vi "Init.vi"(8 "error in":errorcluster, 11 "Session":T1="cam0") -> (0 "error out  - closing camera":errorcluster, 1 "error out":errorcluster, 2 "Success?":bool, 3 "IMAQdx Session OUT":T1, 4 "Gain - READ":dbl, 5 "Message":string, 6 "Exposure Time - READ":dbl, 7 "Device Serial Number":string)   [LabVIEW 2014]
uses:
  <vilib>/userdefined/High Color/IMAQdx.ctl
  <vilib>/vision/driver/IMAQdx.llb/IMAQdx Camera Control Mode.ctl
  <vilib>/vision/driver/IMAQdx.llb/IMAQdx Acquisition Mode.ctl
  <vilib>/vision/driver/NI_Vision_Acquisition_Software.lvlib
  <resource>/objmgr/imaqdx.rc
panel:
  out "ModelName":string
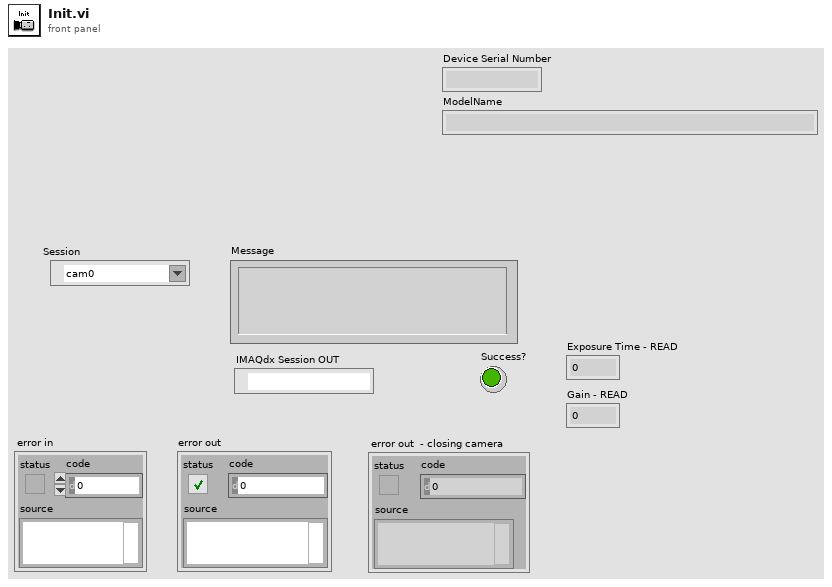
[diagram p1: front panel]
types:
  T1 = typedef "IMAQdx.ctl" = refnum<k21>
  T2 = typedef "NI_Vision_Acquisition_Software.lvlib/IMAQdx Camera Control Mode.ctl" = enum32{"Controller", "Listener"}
  T3 = typedef "NI_Vision_Acquisition_Software.lvlib/IMAQdx Acquisition Mode.ctl" = enum32{"One Shot", "Continuous"}
  T4 = cluster{"Type":u32, "Version":u32, "Flags":u32, "SerialNumberHigh":u32, "SerialNumberLow":u32, "BusType":u32, "InterfaceName":string, "VendorName":string, "ModelName":string, "CameraFileName":string, "CameraAttributeURL":string}[]
  T5 = typedef "NI_Vision_Acquisition_Software.lvlib/IMAQdx Attribute Type.ctl" = enum32{"U32", "I64", "DBL", "String", "Enum", "Bool", "Command"}
  T6 = cluster{"Attribute Type":T5, "Readable":bool, "Writable":bool, "Attribute Name":string}[]
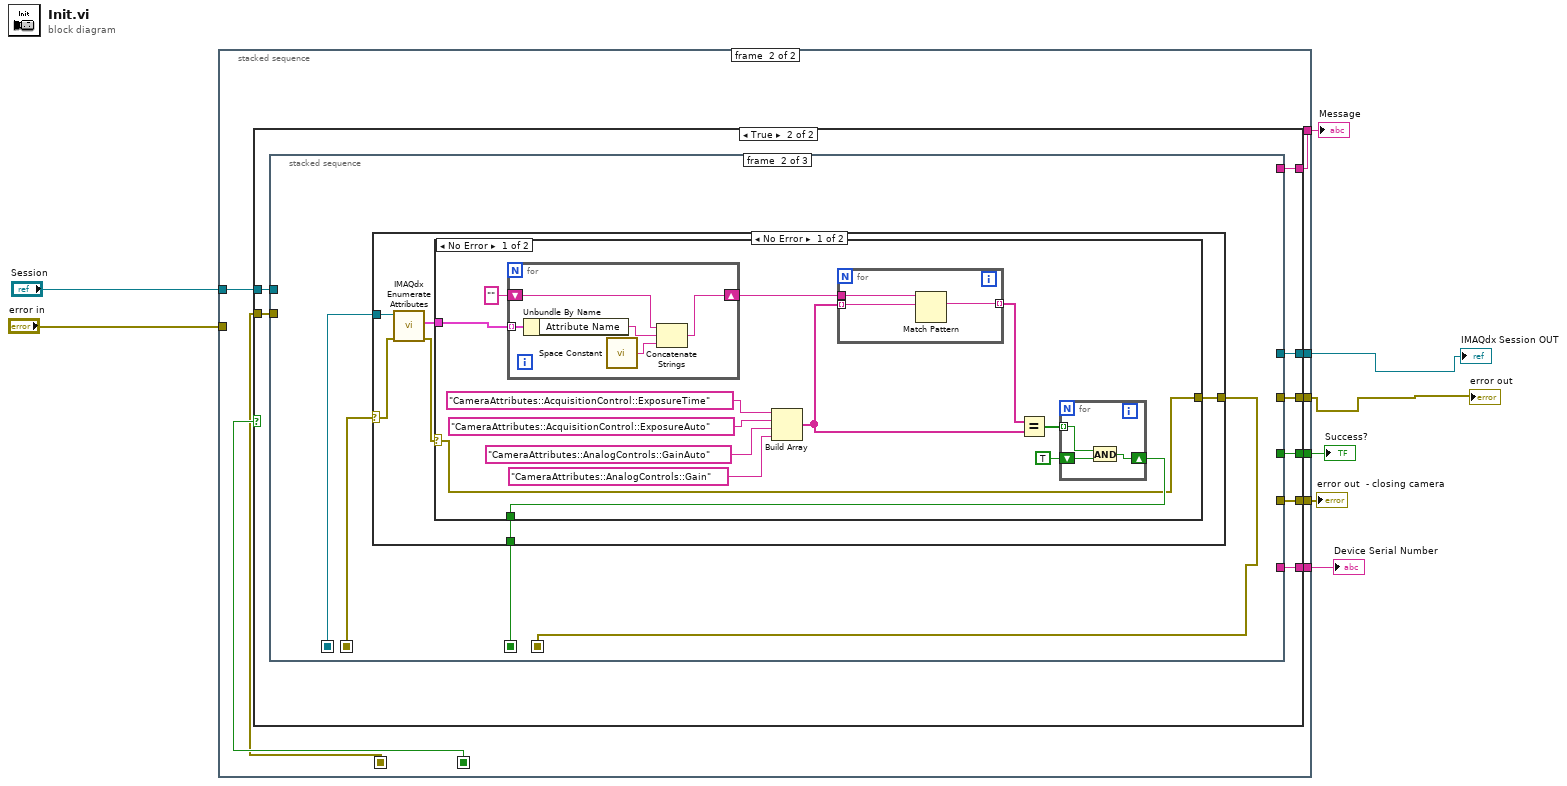
[diagram p0: block diagram]
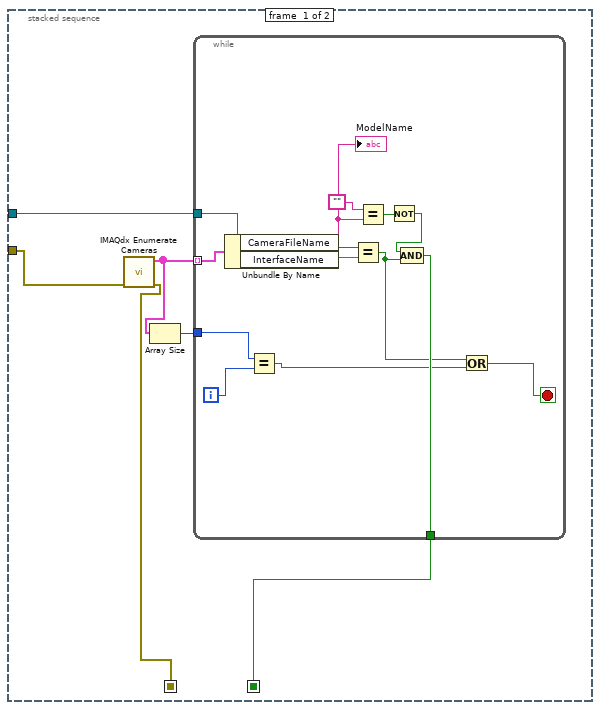
[diagram p2: hidden frame]
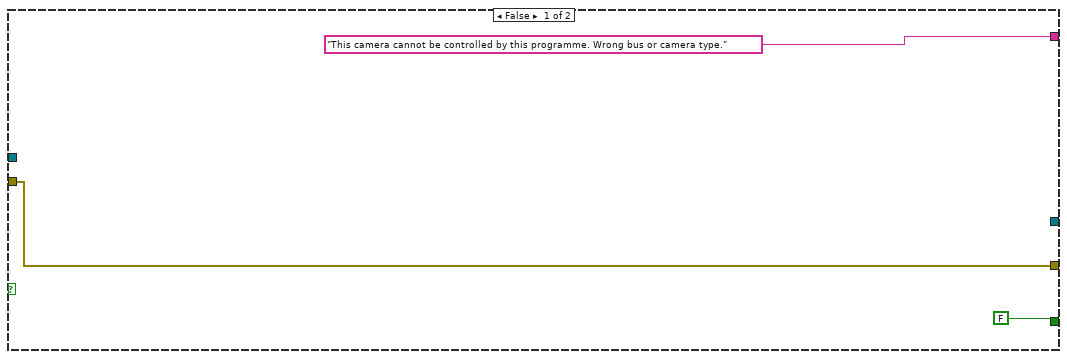
[diagram p3: hidden frame]
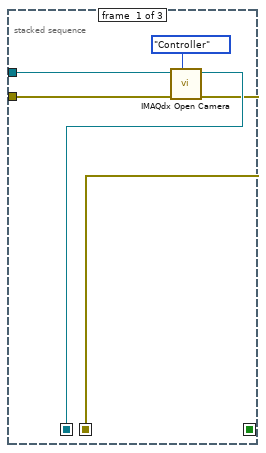
[diagram p4: hidden frame]
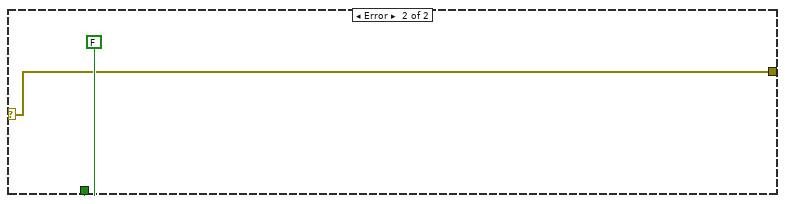
[diagram p5: hidden frame]
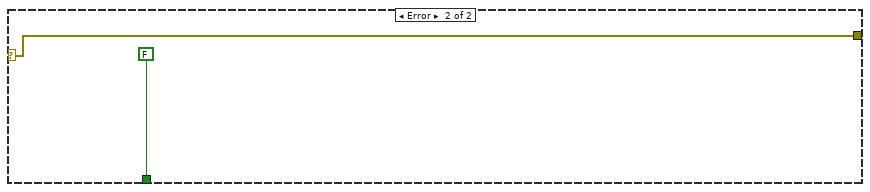
[diagram p6: hidden frame]
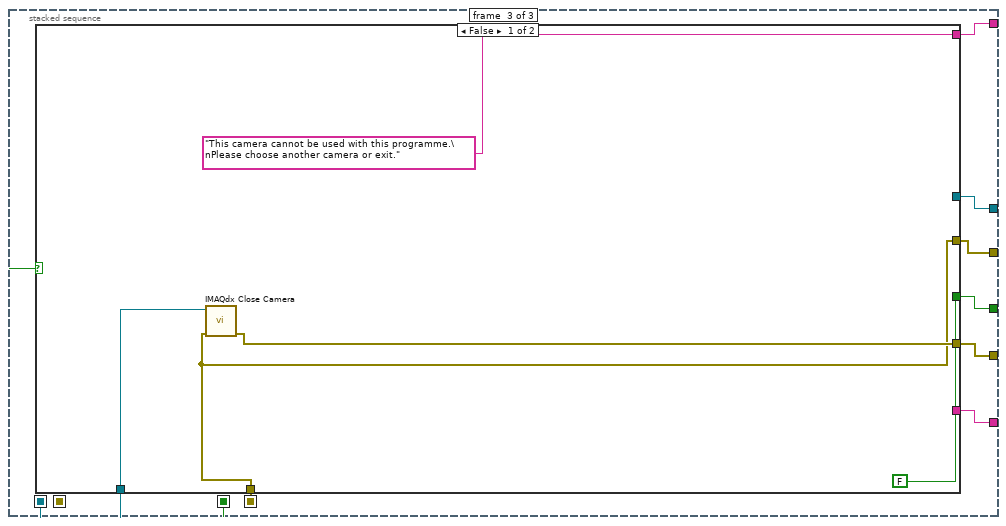
[diagram p7: hidden frame]
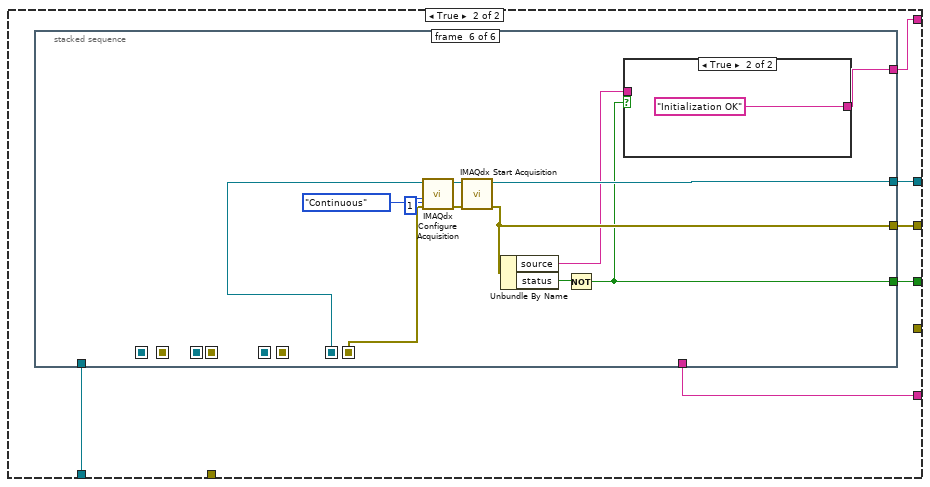
[diagram p8: hidden frame]
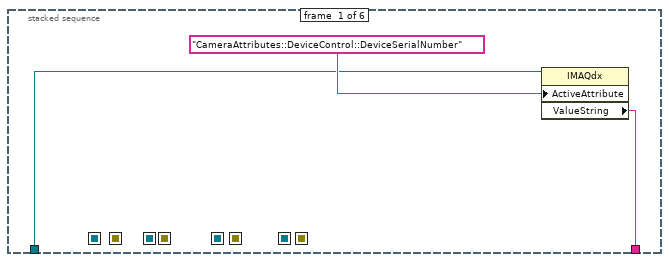
[diagram p9: hidden frame]
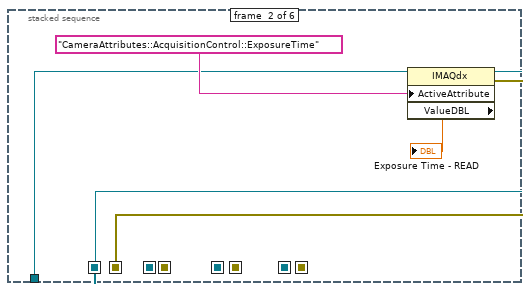
[diagram p10: hidden frame]
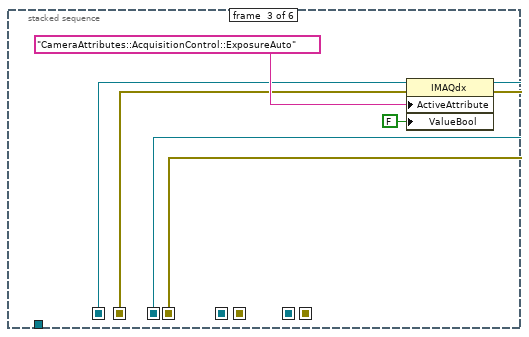
[diagram p11: hidden frame]
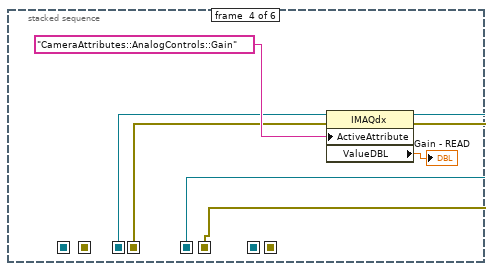
[diagram p12: hidden frame]
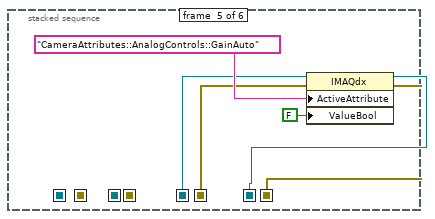
[diagram p13: hidden frame]
diagram:
  n1 = stacked-sequence {
    seq-local: [w13 _] -> [_ w31]
    seq-local: [w9 _] -> [_ w28]
    tunnel: [_ w36] -> w8
    tunnel: [_ w35] -> w2
    tunnel: [_ w30] -> w1
    tunnel: [_ w34] -> w7
    tunnel: "Session" -> [w14 w33]
    tunnel: [_ w32] -> w5
    tunnel: "error in" -> [w10 _]
    tunnel: [_ w29] -> w3
    frame #0 {
      n2 = call <vilib>:"IMAQdx Enumerate Cameras.vi"("error in"=w10) -> ("error out"=w9:errorcluster, "Camera Information Array"=w12:T4)  [unwired: 9 in]
      n3 = Array Size(array=w12) -> (size(s)=w11:i32)
      n4 = while {
        tunnel: w12 -> [w27] mode=indexing
        tunnel: w14 -> [w26]
        tunnel: [w22] -> w13
        tunnel: w11 -> [w23]
        i -> [w24]
        stop <- w20 stop-if-true
        n5 = Unbundle By Name(w27) -> ("CameraFileName"=w19:string, "InterfaceName"=w25:string)
        "ModelName" <- w19
        n6 = Equal?(x=w23, y=w24) -> (x = y?=w21:bool)
        n7 = Equal?(x=w26, y=w25) -> (x = y?=w15:bool)
        n8 = Equal?(x="", y=w19) -> (x = y?=w17:bool)
        n9 = Not(x=w17) -> (.not. x?=w16:bool)
        n10 = Compound Arithmetic op=AND(w16, w15) -> (w22:bool)
        n11 = Or(x=w15, y=w21) -> (x .or. y?=w20:bool)
      }
    }
    frame #1 {
      n12 = case shown="True" w31 {
        tunnel: ["This camera cannot be controlled by this programme. Wrong bus or camera type." ("source") w47] -> w36
        tunnel: [_ w46] -> w35
        tunnel: [FALSE w45] -> w34
        tunnel: w33 -> [_ w44]
        tunnel: [_ w43] -> w32
        tunnel: w28 -> [w38 w42]
        tunnel: [w38 w40] -> w30
        tunnel: [_ w41] -> w29
        frame False {
        }
        frame True {
          n13 = stacked-sequence {
            seq-local: [w50 _ _] -> [_ w54 _]
            seq-local: [w51 _ _] -> [_ w56 w99]
            seq-local: [_ w55 _] -> [_ _ w98]
            seq-local: [_ w53 _] -> [_ _ w92]
            tunnel: [_ _ w97] -> w47
            tunnel: [_ _ w96] -> w46
            tunnel: [_ _ w95] -> w45
            tunnel: w44 -> [w49 _ _]
            tunnel: [_ _ w94] -> w43
            tunnel: w42 -> [w48 _ _]
            tunnel: [_ _ w93] -> w41
            tunnel: [_ _ w91] -> w40
            frame #0 {
              n14 = call <vilib>:"IMAQdx Open Camera.vi"("Camera Control Mode"=IMAQdx_Camera_Control_Mode."Controller", "error in"=w48, "Session In"=w49) -> ("error out"=w50:errorcluster, "Session Out"=w51:T1)  [unwired: 7 in]
            }
            frame #1 {
              n15 = case shown="No Error" w54 {
                selector: w54 -> [w58 w89]
                tunnel: w56 -> [w62 _]
                tunnel: [w60 FALSE] -> w55
                tunnel: [w57 w89] -> w53
                frame No Error {
                  n16 = call <vilib>:"IMAQdx Enumerate Attributes.vi"("error in"=w58, "Session In"=w62) -> ("error out"=w59:errorcluster, "Attribute Information Array"=w61:T6)  [unwired: 7 in, 1 out]
                  n17 = case shown="No Error" w59 {
                    selector: w59 -> [w63 w87]
                    tunnel: w61 -> [w75 _]
                    tunnel: [w65 FALSE] -> w60
                    tunnel: [w63 w87] -> w57
                    frame No Error {
                      n18 = for {
                        tunnel: w75 -> [w86] mode=indexing
                        shift-right: [w83] -> w69
                        shift-left: "" -> [w82]
                        n19 = Unbundle By Name(w86) -> ("Attribute Name"=w85:string)
                        n20 = call <vilib>:"Space Constant.vi"() -> ("String"=w84:string)
                        n21 = Concatenate Strings(w82, w85, w84) -> (w83:string)
                      }
                      n22 = Build Array("CameraAttributes::AcquisitionControl::ExposureTime" ("Attribute Name"), "CameraAttributes::AcquisitionControl::ExposureAuto" ("Attribute Name"), "CameraAttributes::AnalogControls::GainAuto" ("Attribute Name"), "CameraAttributes::AnalogControls::Gain" ("Attribute Name")) -> (w64:string[])
                      n23 = for {
                        tunnel: w69 -> [w81]
                        tunnel: w64 -> [w80] mode=indexing
                        tunnel: [w79] -> w68 mode=indexing
                        n24 = Match Pattern(string=w81, regular expression=w80) -> (match substring=w79:string)  [unwired: 1 in, 3 out]
                      }
                      n25 = Equal?(x=w68, y=w64) -> (x = y?=w67:bool[])
                      n26 = for {
                        tunnel: w67 -> [w78] mode=indexing
                        shift-right: [w76] -> w65
                        shift-left: TRUE -> [w77]
                        n27 = And(x=w78, y=w77) -> (x .and. y?=w76:bool)
                      }
                    }
                    frame Error {
                    }
                  }
                }
                frame Error {
                }
              }
            }
            frame #2 {
              n28 = case shown="False" w98 {
                tunnel: w99 -> [w104 w110]
                tunnel: ["This camera cannot be used with this programme.\nPlease choose another camera or exit." w106] -> w97
                tunnel: [_ w109] -> w96
                tunnel: [w100 w108] -> w91
                tunnel: [FALSE w107] -> w95
                tunnel: [w101 _] -> w94
                tunnel: [_ w105] -> w93
                tunnel: w92 -> [w100 _]
                frame False {
                  n29 = call <vilib>:"IMAQdx Close Camera.vi"("error in"=w100, "Session In"=w104) -> ("error out"=w101:errorcluster)  [unwired: 9 in]
                }
                frame True {
                  n30 = stacked-sequence {
                    seq-local: [_ w115 _ _ _ _] -> [_ _ w121 _ _ _]
                    seq-local: [_ w114 _ _ _ _] -> [_ _ w122 _ _ _]
                    seq-local: [_ _ w120 _ _ _] -> [_ _ _ w128 _ _]
                    seq-local: [_ _ w119 _ _ _] -> [_ _ _ w127 _ _]
                    seq-local: [_ _ _ w126 _ _] -> [_ _ _ _ w134 _]
                    seq-local: [_ _ _ w125 _ _] -> [_ _ _ _ w133 _]
                    seq-local: [_ _ _ _ w132 _] -> [_ _ _ _ _ w141]
                    seq-local: [_ _ _ _ w131 _] -> [_ _ _ _ _ w140]
                    tunnel: w110 -> [w112 w117 _ _ _ _]
                    tunnel: [_ _ _ _ _ w144] -> w109
                    tunnel: [_ _ _ _ _ w143] -> w108
                    tunnel: [_ _ _ _ _ w139] -> w107
                    tunnel: [_ _ _ _ _ w138] -> w106
                    tunnel: [w111 _ _ _ _ _] -> w105
                    frame #0 {
                      n31 = property class="IMAQdx"(reference=w112, "ActiveAttribute"="CameraAttributes::DeviceControl::DeviceSerialNumber" ("Attribute Name")) -> ("ValueString"=w111:string)  [unwired: 1 in, 2 out]
                    }
                    frame #1 {
                      n32 = property class="IMAQdx"(reference=w117, "ActiveAttribute"="CameraAttributes::AcquisitionControl::ExposureTime" ("Attribute Name")) -> (reference out=w114:T1, error out=w115:errorcluster, "ValueDBL"=→"Exposure Time - READ":dbl)  [unwired: 1 in]
                    }
                    frame #2 {
                      n33 = property class="IMAQdx"(reference=w122, error in=w121, "ActiveAttribute"="CameraAttributes::AcquisitionControl::ExposureAuto" ("Attribute Name"), "ValueBool"=FALSE) -> (reference out=w120:T1, error out=w119:errorcluster)
                    }
                    frame #3 {
                      n34 = property class="IMAQdx"(reference=w128, error in=w127, "ActiveAttribute"="CameraAttributes::AnalogControls::Gain") -> (reference out=w126:T1, error out=w125:errorcluster, "ValueDBL"=→"Gain - READ":dbl)
                    }
                    frame #4 {
                      n35 = property class="IMAQdx"(reference=w134, error in=w133, "ActiveAttribute"="CameraAttributes::AnalogControls::GainAuto" ("Attribute Name"), "ValueBool"=FALSE) -> (reference out=w132:T1, error out=w131:errorcluster)
                    }
                    frame #5 {
                      n36 = call <vilib>:"IMAQdx Configure Acquisition.vi"("error in"=w140, "Number of Buffers"=1, "Continuous?"=IMAQdx_Acquisition_Mode."Continuous", "Session In"=w141) -> ("error out"=w147:errorcluster, "Session Out"=w146:T1)  [unwired: 6 in]
                      n37 = call <vilib>:"IMAQdx Start Acquisition.vi"("error in"=w147, "Session In"=w146) -> ("error out"=w143:errorcluster, "Session Out"=w144:T1)  [unwired: 8 in]
                      n38 = Unbundle By Name(w143) -> ("source"=w137:string, "status"=w142:bool)
                      n39 = Not(x=w142) -> (.not. x?=w139:bool)
                      n40 = case shown="True" w139 {
                        tunnel: [w149 "Initialization OK"] -> w138
                        tunnel: w137 -> [w149 _]
                        frame False {
                        }
                        frame True {
                        }
                      }
                    }
                  }
                }
              }
            }
          }
        }
      }
    }
  }
  "Message" <- w8
  "Success?" <- w7
  "error out  - closing camera" <- w5
  "Device Serial Number" <- w3
  "error out" <- w1
  "IMAQdx Session OUT" <- w2
